vi "DllFxpReciprocalTemp.vi"(6 "ready for output":bool, 9 "input valid":bool, 11 "x":fxp<+/-,16,1>) -> (1 "output valid":bool, 2 "overflow?":bool, 3 "1/x":fxp<+/-,16,16>, 4 "ready for input":bool)   [LabVIEW 2017]
uses:
  <vilib>/rvi/FXPMathLib/FxpDiv/subVIs/nifxpmath_Div_SimConfig.ctl
  <vilib>/rvi/FXPMathLib/FxpDiv/simVIs/DllFxpDivTemp_sub.vi
  <vilib>/rvi/FXPMathLib/FxpDiv/XNode/nifxpmath_Div.xnode
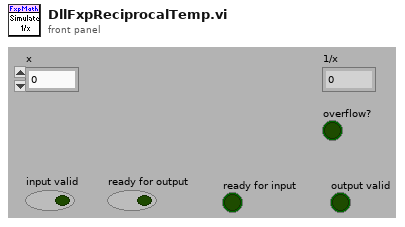
[diagram p1: front panel]
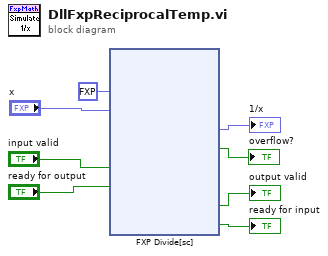
[diagram p0: block diagram]
diagram:
  n1 = xnode "FXP Divide[sc]"("x"=fxp<+,1,1> 1.0, "y"="x", "input valid"="input valid", "ready for output (T)"="ready for output") -> ("x/y"=→"1/x":fxp<+/-,16,16>, "operation overflow"=→"overflow?":bool, "output valid"=→"output valid":bool, "ready for input"=→"ready for input":bool)
